vi "CTRE_PigeonIMU_ConfigGetSlot.vi"(6 "timeoutMs":i32=50, 8 "error in":errorcluster, 11 "PigeonIMUDevRef":T3={"DeviceStatus"={"status"=FALSE, "code"=0, "source"=""}, "Device Number"=0, "Type"=352321536, "Device ID"=0, "Handle"=0, "UsageFrame"=0, "Library Path"=path ""} {"Type" items=["CAN"=352321536, "TalonSRX"=33554432]}) -> (0 "error out":errorcluster, 2 "Pigeon Config Parameters":T1, 3 "PigeonIMUDevRef":T3={"DeviceStatus"={"status"=FALSE, "code"=0, "source"=""}, "Device Number"=0, "Type"=352321536, "Device ID"=0, "Handle"=0, "UsageFrame"=0, "Library Path"=path ""} {"Type" items=["CAN"=352321536, "TalonSRX"=33554432]})   [LabVIEW 2019]
doc: "Gets all persistant settings"
uses:
  <vilib>/Rock Robotics/WPI/ThirdParty/Phoenix-LabVIEW/Pigeon IMU/CTRE_PigeonIMU_DeviceRef.ctl
  <vilib>/Rock Robotics/WPI/ThirdParty/Phoenix-LabVIEW/Pigeon IMU/CTRE_PigeonIMU_ConnectionType.ctl
  <vilib>/Rock Robotics/WPI/ThirdParty/Phoenix-LabVIEW/Pigeon IMU/CTRE_PigeonIMU_Configurables.ctl
  <vilib>/Rock Robotics/WPI/ThirdParty/Phoenix-LabVIEW/Controls/CTRE_Phoenix_CustomParamConfiguration.ctl
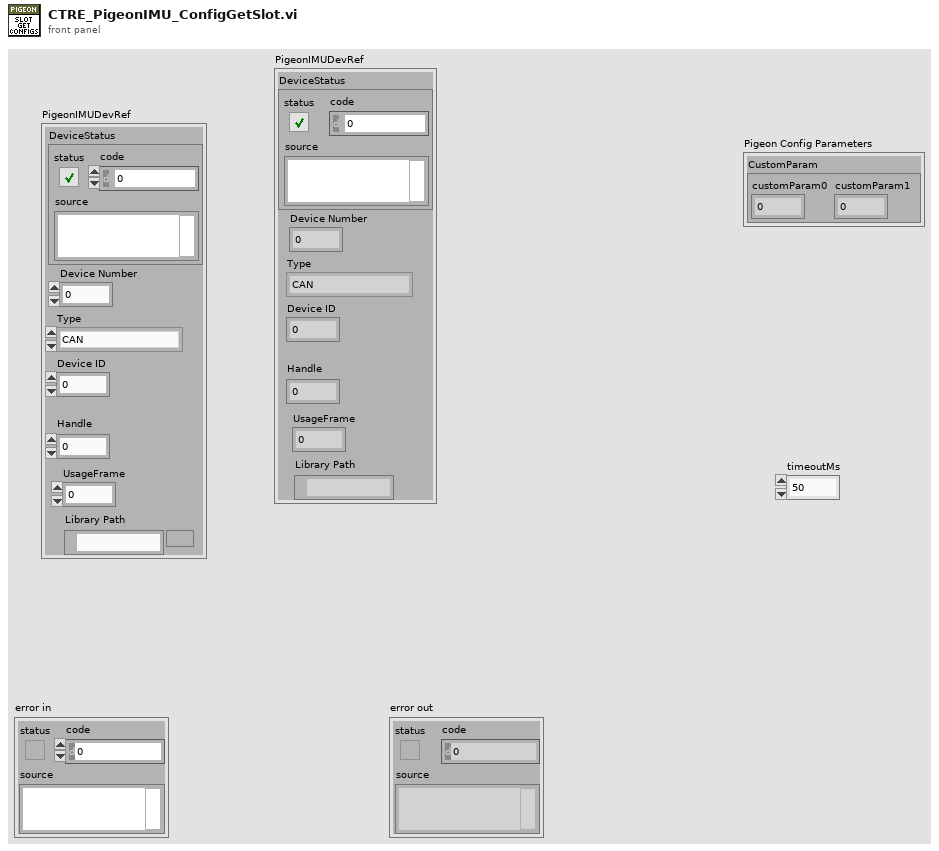
[diagram p1: front panel]
types:
  T1 = typedef "CTRE_PigeonIMU_Configurables.ctl" = cluster{"CustomParam":T2}
  T2 = typedef "CTRE_Phoenix_CustomParamConfiguration.ctl" = cluster{"customParam0":i32, "customParam1":i32}
  T3 = typedef "CTRE_PigeonIMU_DeviceRef.ctl" = cluster{"DeviceStatus":errorcluster, "Device Number":u8, "Type":T4, "Device ID":u32, "Handle":u64, "UsageFrame":u32, "Library Path":path}
  T4 = typedef "CTRE_PigeonIMU_ConnectionType.ctl" = u32
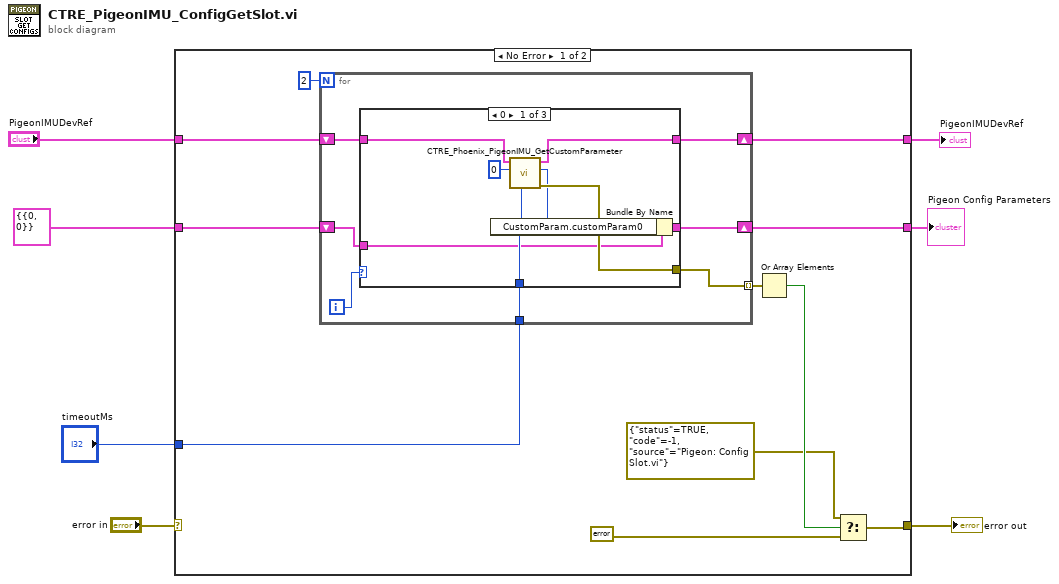
[diagram p0: block diagram]
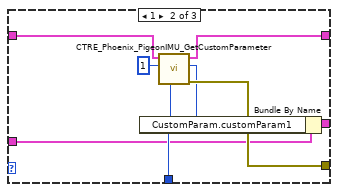
[diagram p2: hidden frame]
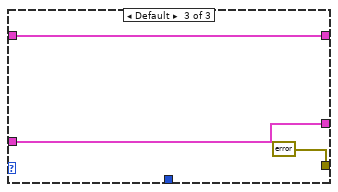
[diagram p3: hidden frame]
diagram:
  n1 = case shown="No Error" "error in" {
    selector: "error in" -> [_ w47]
    tunnel: [w13 w47] -> w6
    tunnel: "PigeonIMUDevRef" -> [w18 w46]
    tunnel: "timeoutMs" -> [w15 _]
    tunnel: [w17 w46] -> w3
    tunnel: T1 {"CustomParam"={"customParam0"=0, "customParam1"=0}} ("Pigeon Config Parameters 2") -> [w16 w45]
    tunnel: [w8 w45] -> w2
    frame No Error {
      n2 = for {
        N: 2 -> [_]
        shift-right: [w23] -> w17
        shift-left: w18 -> [w24]
        tunnel: [w21] -> w14 mode=indexing
        tunnel: w15 -> [w20]
        shift-right: [w19] -> w8
        shift-left: w16 -> [w22]
        i -> [w25]
        n3 = case shown="0" w25 {
          tunnel: w24 -> [w33 w41 w44]
          tunnel: [w32 w40 w44] -> w23
          tunnel: w22 -> [w28 w36 w42]
          tunnel: [w31 w39 errorcluster {"status"=FALSE, "code"=0, "source"=""} ("error out")] -> w21
          tunnel: w20 -> [w30 w38 _]
          tunnel: [w26 w37 w42] -> w19
          frame 0 {
            n4 = call <vilib>:"CTRE_Phoenix_PigeonIMU_GetCustomParameter.vi"("timeoutMs"=w30, "paramIndex"=0, "PigeonIMUDevRef"=w33) -> ("error out"=w31:errorcluster, "readValue"=w27:i32, "PigeonIMUDevRef"=w32:T3)  [unwired: 6 in]
            n5 = Bundle By Name(cluster=w28, "CustomParam.customParam0"=w27) -> (w26:T1)
          }
          frame 1 {
            n6 = call <vilib>:"CTRE_Phoenix_PigeonIMU_GetCustomParameter.vi"("timeoutMs"=w38, "paramIndex"=1, "PigeonIMUDevRef"=w41) -> ("error out"=w39:errorcluster, "readValue"=w34:i32, "PigeonIMUDevRef"=w40:T3)  [unwired: 6 in]
            n7 = Bundle By Name(cluster=w36, "CustomParam.customParam1"=w34) -> (w37:T1)
          }
          frame Default {
          }
        }
      }
      n8 = Or Array Elements(Boolean array=w14) -> (logical OR=w11:bool)
      n9 = Select(t=errorcluster {"status"=TRUE, "code"=-1, "source"="Pigeon: Config Slot.vi"} ("error out"), s=w11, f=errorcluster {"status"=FALSE, "code"=0, "source"=""} ("error out")) -> (s? t:f=w13:errorcluster)
    }
    frame Error {
    }
  }
  "error out" <- w6
  "PigeonIMUDevRef" <- w3
  "Pigeon Config Parameters" <- w2
